vi "Main.vi"(11 "Module Admin":refnum<class "Delacor_lib_QMH_Cloneable Module Admin.lvclass">) -> ()   [LabVIEW 2024, in "Clon.lvlib"]
doc: "This template is based off of the Queued Message Handler design pattern and the Queued Message Handler project template that ships with LabVIEW.\n\nThe main difference is that the queue is private to this module and communication between modules is performed via Broadcast and Request events.\n\nRequest events are wrapped in public API methods and are handled in the Event Handling Loop (EHL) of this VI. Any module can register for Broadcast events sent by this module. The EHL generates messages based on user interface actions.\n\nThe Message Handling Loop (MHL) processes messages generated by the EHL, or by other messages. The messages are string values, so new messages can be added easily to the Message Cases case structure in the MHL. Each message cluster can also provide an optional value for Message Data, which is a variant that can be converted to whatever message-specific data is required.\n_____\nBased on DQMH Dev Tools: Project Template 7.1.0.1503."
uses:
  Clon.lvlib
  <vilib>/Delacor/Delacor QMH/Libraries/Cloneable Module Admin_class/Delacor_lib_QMH_Cloneable Module Admin.lvclass
  Module Data--cluster.ctl
  <vilib>/Delacor/Delacor QMH/Libraries/Message Queue_class/Delacor_lib_QMH_Message Queue.lvclass/Delacor_lib_QMH_Message Queue.ctl
  <vilib>/Delacor/Delacor QMH/Libraries/Cloneable Module Admin_class/Delacor_lib_QMH_Cloneable Module Admin.lvclass/Delacor_lib_QMH_Cloneable Module Admin.ctl
  Stop Argument--cluster.ctl
  <vilib>/Delacor/Delacor QMH/Libraries/Module Admin_class/Delacor_lib_QMH_Module Admin.lvclass/Delacor_lib_QMH_Module Admin.ctl
  Set Volts Argument--cluster.ctl
  <vilib>/Utility/miscctls.llb/LVPointTypeDef.ctl
  <vilib>/Delacor/Delacor QMH/Libraries/Message Queue_class/Delacor_lib_QMH_Enqueue Message (Single).vi
  <vilib>/Delacor/Delacor QMH/Libraries/Cloneable Module Admin_class/Delacor_lib_QMH_Get Module ID.vi
  <vilib>/Delacor/Delacor QMH/Libraries/Module Admin_class/Delacor_lib_QMH_Get External Launch.vi
  <vilib>/Delacor/Delacor QMH/Libraries/Message Queue_class/Delacor_lib_QMH_Message Queue.lvclass
panel:
  out "Meter":dbl(knob) scale=0.0..10.0
  out "error out":errorcluster
  out "Status":string
  in  "Simulate EHL Error":bool
  in  "Simulate MHL Error":bool
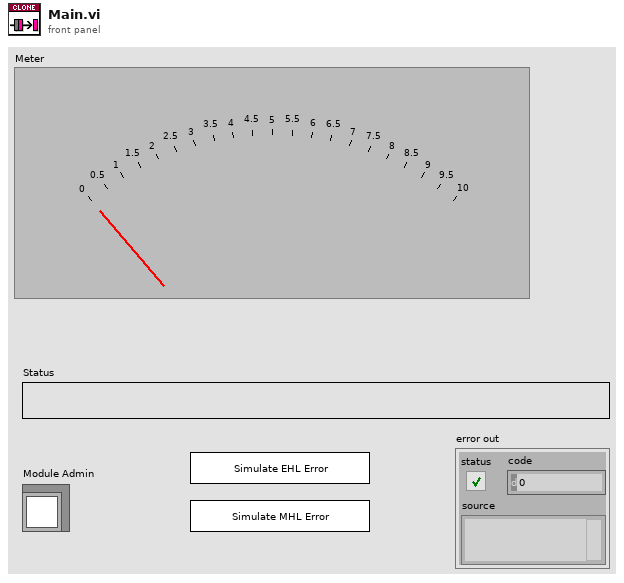
[diagram p1: front panel]
types:
  T1 = typedef "Clon.lvlib/Request Events--cluster.ctl" = cluster{"Stop Module":refnum<user-event>, "Show Panel":refnum<user-event>, "Hide Panel":refnum<user-event>, "Show Diagram":refnum<user-event>, "Get Module Execution Status":refnum<user-event>, "Set Volts":refnum<user-event>}
  T2 = typedef "Clon.lvlib/Module Data--cluster.ctl" = cluster{"Status":string}
  T3 = enum32{"invalid lock state", "Not Locked", "Locked (No Password)", "Password-protected"}
  T4 = typedef "Clon.lvlib/Stop Argument--cluster.ctl" = cluster{"Module ID":i32, "Origin":string, "Exit via Stop Module Req?":bool, "Wait for Module to stop?":bool}
  T5 = typedef "Clon.lvlib/Set Volts Argument--cluster.ctl" = cluster{"Module ID":i32, "Volts":dbl}
  T6 = typedef "LVPointTypeDef.ctl" = cluster{"Horizontal":i16, "Vertical":i16}
  T7 = enum32{"Invalid", "Standard", "Closed", "Hidden", "Minimized", "Maximized"}
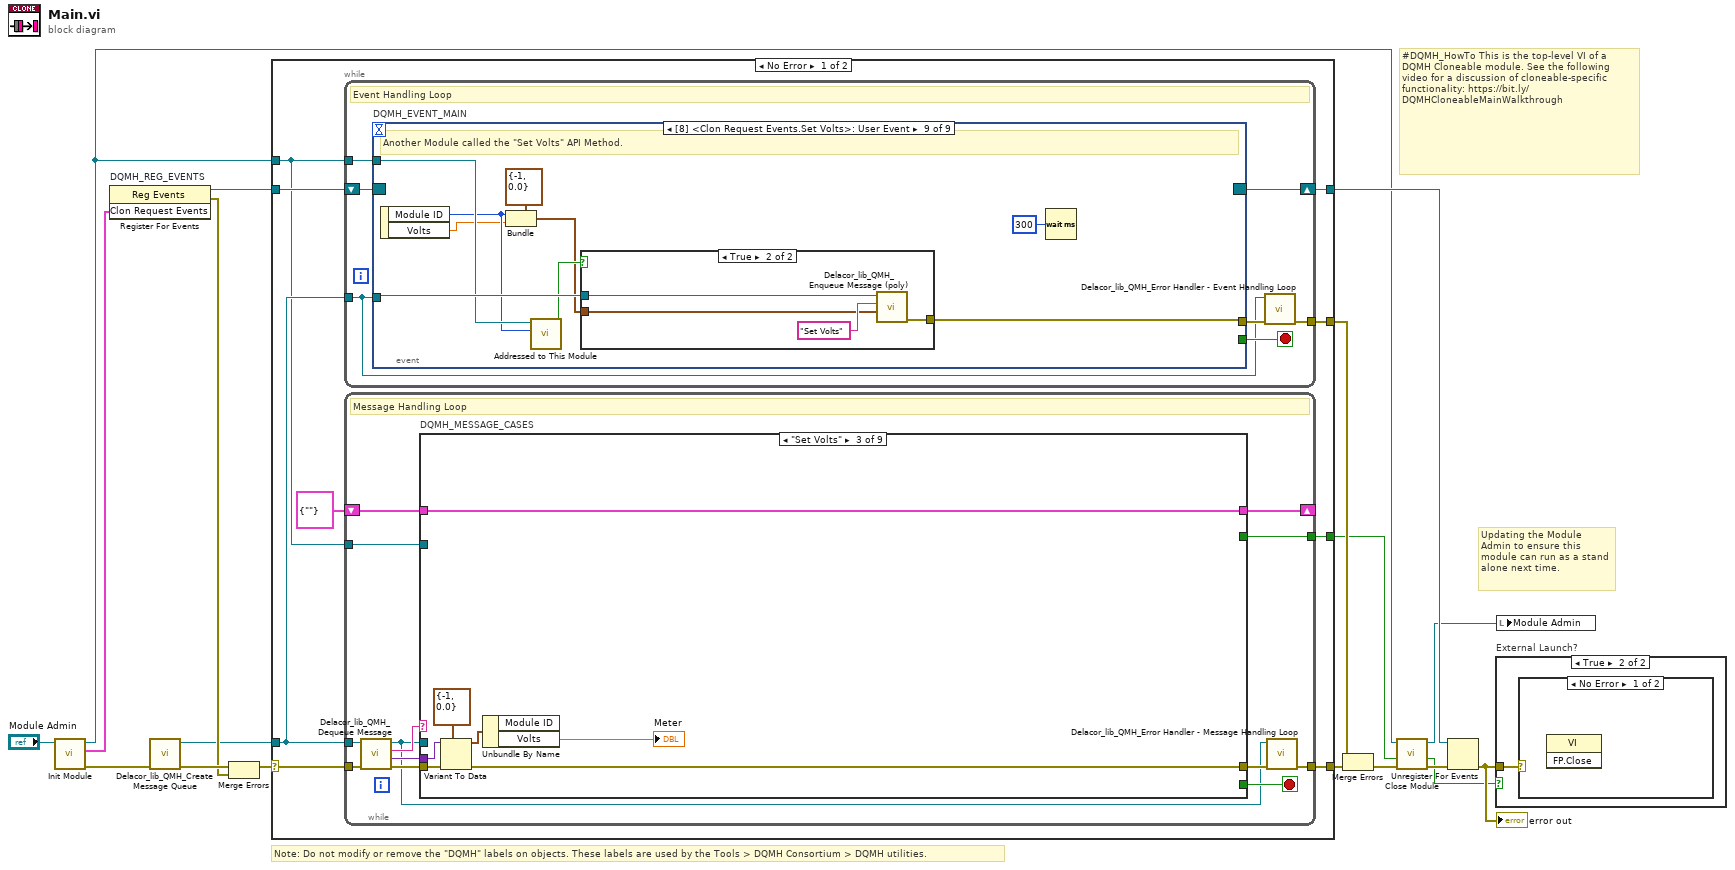
[diagram p0: block diagram]
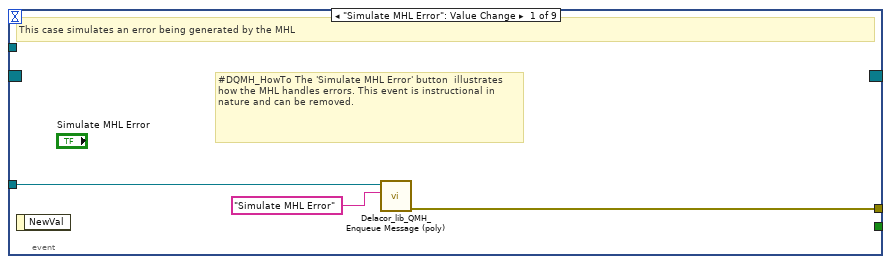
[diagram p2: hidden frame]
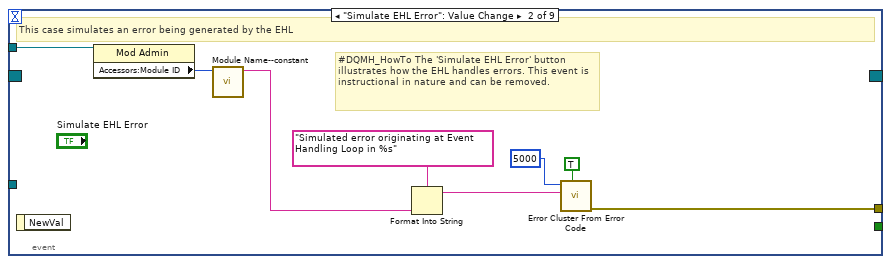
[diagram p3: hidden frame]
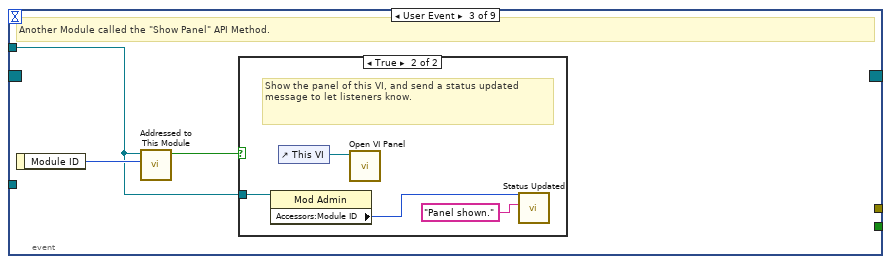
[diagram p4: hidden frame]
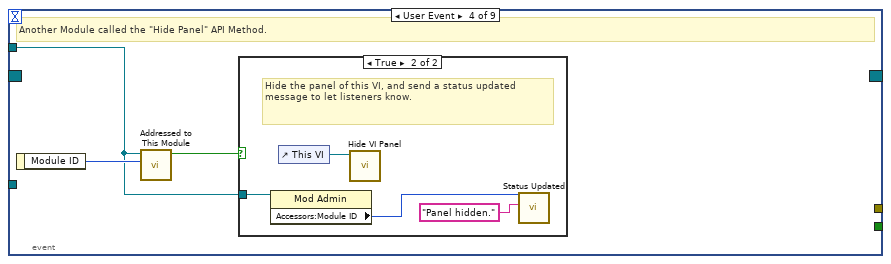
[diagram p6: hidden frame]
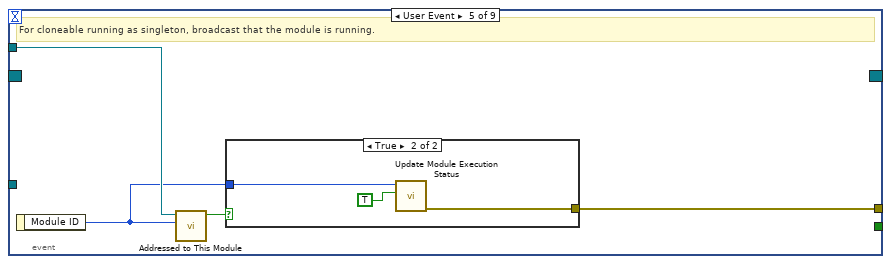
[diagram p8: hidden frame]
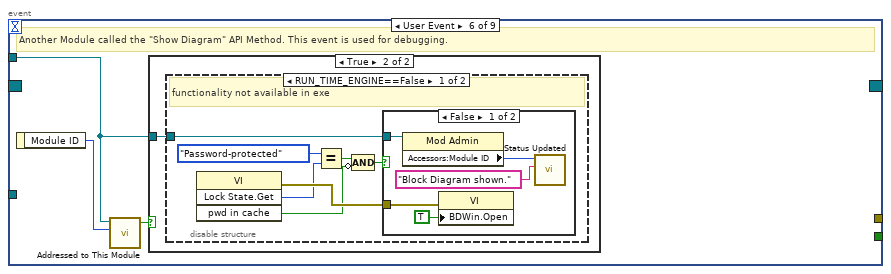
[diagram p10: hidden frame]
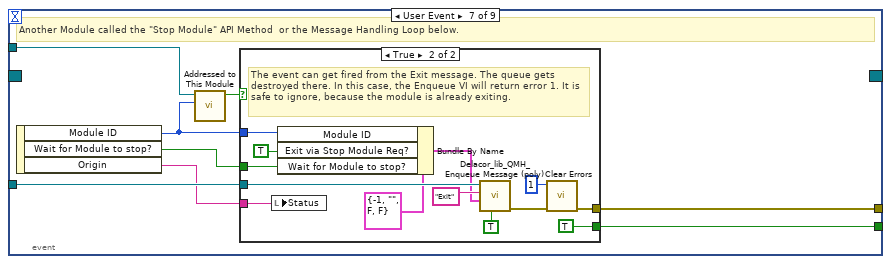
[diagram p14: hidden frame]
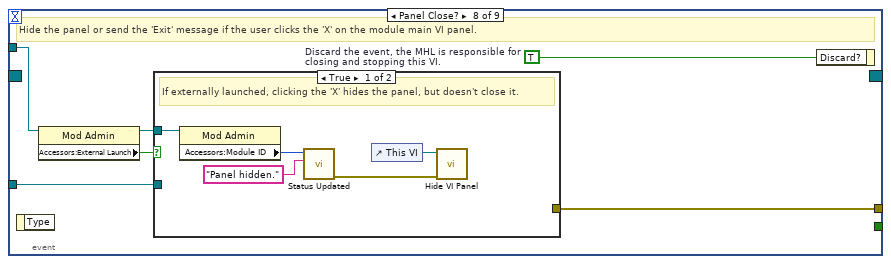
[diagram p16: hidden frame]
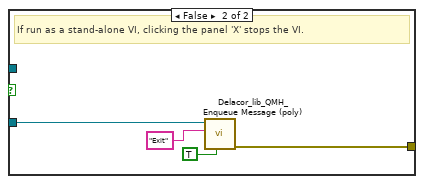
[diagram p17: hidden frame]
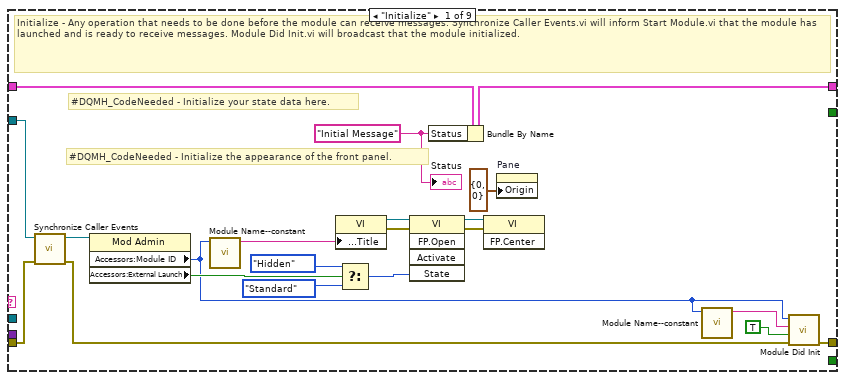
[diagram p19: hidden frame]
diagram:
  # "#DQMH_HowTo This is the top-level VI of a DQMH Cloneable module. See the following video for a discussion of cloneable-specific functionality: https://bit.ly/DQMHCloneableMainWalkthrough"
  # "Note: Do not modify or remove the \"DQMH\" labels on objects. These labels are used by the Tools > DQMH Consortium > DQMH utilities."
  # "Updating the Module Admin to ensure this module can run as a stand alone next time."
  n1 = call "Init Module.vi"("Cloneable Module Admin in"="Module Admin") -> ("error out"=w15:errorcluster, "Clon Request Events"=w7:T1, "Cloneable Module Admin out"=w4:refnum<class "Delacor_lib_QMH_Cloneable Module Admin.lvclass">)  [unwired: 8 in]
  n2 = register-events "DQMH_REG_EVENTS"(w7) -> (reference out=w8:refnum<event-registration>, error out=w10:errorcluster)  [unwired: 2 in]
  n3 = call <vilib>:"Delacor_lib_QMH_Create Message Queue.vi"("error in"=w15) -> ("error out"=w12:errorcluster, "Message Queue"=w6:refnum<class "Delacor_lib_QMH_Message Queue.lvclass">)  [unwired: 9 in]
  n4 = Merge Errors(w12, w10) -> (w11:errorcluster)
  n5 = case shown="No Error" w11 {
    selector: w11 -> [w25 w247]
    tunnel: [w27 w246] -> w16
    tunnel: [w24 w245] -> w9
    tunnel: w8 -> [w22 w245]
    tunnel: w6 -> [w21 w238]
    tunnel: [w26 _] -> w17
    tunnel: w4 -> [w20 w241]
    tunnel: [w19 _] -> w2
    frame No Error {
      n6 = while {
        tunnel: w21 -> [w28]
        shift-right: [w31] -> w24
        shift-left: w22 -> [w32]
        tunnel: [w33] -> w26
        tunnel: w20 -> [w29]
        stop <- w30 stop-if-true
        # "Event Handling Loop"
        n7 = event "DQMH_EVENT_MAIN" shown="[8] <Clon Request Events.Set Volts>: User Event" {
          selector: w32 -> [_ _ _ _ _ _ _ _ _]
          dyn-events: [_ _ _ _ _ _ _ _ _] -> w31
          timeout: _ -> [_ _ _ _ _ _ _ _ _]
          tunnel: [_ _ _ _ _ _ w86 _ _] -> w30
          tunnel: w28 -> [w36 _ _ _ _ _ w89 w106 w127]
          tunnel: [w37 w45 _ _ w63 _ w90 w109 w120] -> w34
          tunnel: w29 -> [_ w44 w46 w53 w61 w67 w88 w107 w125]
          event "Simulate MHL Error": Value Change {
            # "#DQMH_HowTo The 'Simulate MHL Error' button  illustrates how the MHL handles errors. This event is instructional in nature and can be removed."
            # "This case simulates an error being generated by the MHL"
            n8 = event-data() -> ()  [unwired: 1 in, 1 out]
            n9 = call-poly <vilib>:"Delacor_lib_QMH_Enqueue Message (poly).vi"("Message"="Simulate MHL Error", "Message Queue in"=w36) -> ("error out"=w37:errorcluster)  [unwired: 8 in, 1 out]
          }
          event "Simulate EHL Error": Value Change {
            # "#DQMH_HowTo The 'Simulate EHL Error' button  illustrates how the EHL handles errors. This event is instructional in nature and can be removed."
            # "This case simulates an error being generated by the EHL"
            n10 = event-data() -> ()  [unwired: 1 in, 1 out]
            n11 = property on="Property Node" class="Mod Admin"(reference=w44) -> ("Accessors:Module ID"=w43:i32)  [unwired: 1 in, 2 out]
            n12 = call "Module Name--constant.vi"("Module ID"=w43) -> ("Module Name"=w38:string)  [unwired: 10 in]
            n13 = Format Into String(format string="Simulated error originating at Event Handling Loop in %s", w38) -> (resulting string=w41:string)  [unwired: 2 in, 1 out]
            n14 = call <vilib>:"Error Cluster From Error Code.vi"("show call chain? (False)"=TRUE, "error message (\"\")"=w41, "error code (0)"=5000) -> ("error out"=w45:errorcluster)  [unwired: 6 in]
          }
          event User Event {
            # "Another Module called the \"Show Panel\" API Method."
            n15 = event-data() -> ("Module ID"=w47:i32)  [unwired: 1 in]
            n16 = call "Addressed to This Module.vi"("Module ID from Argument"=w47, "Module Admin"=w46) -> ("Addressed to this instance?"=w48:bool)  [unwired: 8 in, 1 out]
            n17 = case shown="True" w48 {
              tunnel: w46 -> [_ w50]
              frame False {
              }
              frame True {
                # "Show the panel of this VI, and send a status updated message to let listeners know."
                n18 = property on="Property Node" class="Mod Admin"(reference=w50) -> ("Accessors:Module ID"=w49:i32)  [unwired: 1 in, 2 out]
                n19 = control-ref of="This VI"() -> (w52:refnum<vi>)
                n20 = call "Open VI Panel.vi"("VI"=w52) -> ()  [unwired: 10 in, 1 out]
                n21 = call "Status Updated.vi"("Status"="Panel shown." ("format string"), "Module ID"=w49) -> ()  [unwired: 9 in, 1 out]
              }
            }
          }
          event User Event {
            # "Another Module called the \"Hide Panel\" API Method."
            n22 = event-data() -> ("Module ID"=w54:i32)  [unwired: 1 in]
            n23 = call "Addressed to This Module.vi"("Module ID from Argument"=w54, "Module Admin"=w53) -> ("Addressed to this instance?"=w55:bool)  [unwired: 8 in, 1 out]
            n24 = case shown="True" w55 {
              tunnel: w53 -> [_ w57]
              frame False {
              }
              frame True {
                # "Hide the panel of this VI, and send a status updated message to let listeners know."
                n25 = property on="Property Node" class="Mod Admin"(reference=w57) -> ("Accessors:Module ID"=w56:i32)  [unwired: 1 in, 2 out]
                n26 = control-ref of="This VI"() -> (w59:refnum<vi>)
                n27 = call "Hide VI Panel.vi"("VI"=w59) -> ()  [unwired: 10 in, 1 out]
                n28 = call "Status Updated.vi"("Status"="Panel hidden." ("format string"), "Module ID"=w56) -> ()  [unwired: 9 in, 1 out]
              }
            }
          }
          event User Event {
            # "For cloneable running as singleton, broadcast that the module is running."
            n29 = event-data() -> ("Module ID"=w60:i32)  [unwired: 1 in]
            n30 = call "Addressed to This Module.vi"("Module ID from Argument"=w60, "Module Admin"=w61) -> ("Addressed to this instance?"=w62:bool)  [unwired: 8 in, 1 out]
            n31 = case shown="True" w62 {
              tunnel: [_ w66] -> w63
              tunnel: w60 -> [_ w65]
              frame False {
              }
              frame True {
                n32 = call "Update Module Execution Status.vi"("Running?"=TRUE, "Module ID"=w65) -> ("error out"=w66:errorcluster)  [unwired: 9 in]
              }
            }
          }
          event User Event {
            # "Another Module called the \"Show Diagram\" API Method. This event is used for debugging."
            n33 = event-data() -> ("Module ID"=w68:i32)  [unwired: 1 in]
            n34 = call "Addressed to This Module.vi"("Module ID from Argument"=w68, "Module Admin"=w67) -> ("Addressed to this instance?"=w69:bool)  [unwired: 8 in, 1 out]
            n35 = case shown="True" w69 {
              tunnel: w67 -> [_ w70]
              frame False {
              }
              frame True {
                n36 = disable-structure shown="RUN_TIME_ENGINE==False" {
                  disable-tunnel: w70 -> [w71 _]
                  frame condition #0 (active) {
                    # "functionality not available in exe"
                    n37 = invoke on="Invoke Node" class="VI" method="Lock State.Get"() -> (error out=w77:errorcluster, "Get Lock State"=w76:T3, "pwd in cache"=w73:bool)  [unwired: 4 in, 1 out]
                    n38 = Equal?(x=T3."Password-protected", y=w76) -> (x = y?=w74:bool)
                    n39 = Compound Arithmetic op=AND(w74, invert w73) -> (w72:bool)
                    n40 = case shown="False" w72 {
                      tunnel: w77 -> [w82 _]
                      tunnel: w71 -> [w79 _]
                      frame False {
                        n41 = property on="Property Node" class="Mod Admin"(reference=w79) -> ("Accessors:Module ID"=w78:i32)  [unwired: 1 in, 2 out]
                        n42 = property on="Property Node" class="VI"(error in=w82, "BDWin.Open"=TRUE ("Block Diagram Window:Open")) -> ()  [unwired: 1 in, 2 out]
                        n43 = call "Status Updated.vi"("Status"="Block Diagram shown." ("format string"), "Module ID"=w78) -> ()  [unwired: 9 in, 1 out]
                      }
                      frame True {
                        # "Password-protected VI, and the password is not in the cache. Do not show the diagram."
                      }
                    }
                  }
                  frame condition #1 {
                  }
                }
              }
            }
          }
          event User Event {
            # "Another Module called the \"Stop Module\" API Method  or the Message Handling Loop below."
            n44 = event-data() -> ("Module ID"=w84:i32, "Wait for Module to stop?"=w85:bool, "Origin"=w83:string)  [unwired: 1 in]
            n45 = call "Addressed to This Module.vi"("Module ID from Argument"=w84, "Module Admin"=w88) -> ("Addressed to this instance?"=w87:bool)  [unwired: 8 in, 1 out]
            n46 = case shown="True" w87 {
              tunnel: [_ w102] -> w90
              tunnel: w89 -> [_ w98]
              tunnel: [_ TRUE] -> w86
              tunnel: w85 -> [_ w93]
              tunnel: w84 -> [_ w95]
              tunnel: w83 -> [_ w91]
              frame False {
              }
              frame True {
                # "The event can get fired from the Exit message. The queue gets destroyed there. In this case, the Enqueue VI will return error 1. It is safe to ignore, because the module is already exiting."
                n47 = local write "Status"(w91) -> ()
                n48 = Bundle By Name(cluster=T4 {"Module ID"=-1, "Origin"="", "Exit via Stop Module Req?"=FALSE, "Wait for Module to stop?"=FALSE} ("Stop Argument"), "Module ID"=w95, "Exit via Stop Module Req?"=TRUE, "Wait for Module to stop?"=w93) -> (w92:T4)
                n49 = call-poly <vilib>:"Delacor_lib_QMH_Enqueue Message (poly).vi"("Priority Message? (F)"=TRUE, "Message Data"=w92, "Message"="Exit", "Message Queue in"=w98) -> ("error out"=w103:errorcluster)  [unwired: 6 in, 1 out]
                n50 = call <vilib>:"Clear Errors.vi"("error in (no error)"=w103, "specific error code to clear (0: all)"=1) -> ("error out"=w102:errorcluster)  [unwired: 4 in, 1 out]
              }
            }
          }
          event Panel Close? {
            w108 = TRUE  # Discard the event, the MHL is responsible for closing and stopping this VI.
            # "Hide the panel or send the 'Exit' message if the user clicks the 'X' on the module main VI panel."
            n51 = event-data() -> ()  [unwired: 1 in, 1 out]
            n52 = property on="Property Node" class="Mod Admin"(reference=w107) -> (reference out=w104:refnum<class "Delacor_lib_QMH_Cloneable Module Admin.lvclass">, "Accessors:External Launch"=w105:bool)  [unwired: 1 in, 1 out]
            n53 = case shown="True" w105 {
              tunnel: w106 -> [_ w117]
              tunnel: [_ w118] -> w109
              tunnel: w104 -> [w112 _]
              frame True {
                # "If externally launched, clicking the 'X' hides the panel, but doesn't close it."
                n54 = property on="Property Node" class="Mod Admin"(reference=w112) -> ("Accessors:Module ID"=w111:i32)  [unwired: 1 in, 2 out]
                n55 = call "Status Updated.vi"("Status"="Panel hidden." ("format string"), "Module ID"=w111) -> ("error out"=w110:errorcluster)  [unwired: 9 in]
                n56 = control-ref of="This VI"() -> (w114:refnum<vi>)
                n57 = call "Hide VI Panel.vi"("error in"=w110, "VI"=w114) -> ()  [unwired: 9 in, 1 out]
              }
              frame False {
                # "If run as a stand-alone VI, clicking the panel 'X' stops the VI."
                n58 = call-poly <vilib>:"Delacor_lib_QMH_Enqueue Message (poly).vi"("Priority Message? (F)"=TRUE, "Message"="Exit", "Message Queue in"=w117) -> ("error out"=w118:errorcluster)  [unwired: 7 in, 1 out]
              }
            }
            n59 = event-data ("Event Filter Node")("Discard?"=w108) -> ()  [unwired: 1 in, 1 out]
          }
          event User Event {
            # "Another Module called the \"Set Volts\" API Method."
            n60 = event-data() -> ("Module ID"=w122:i32, "Volts"=w121:dbl)  [unwired: 1 in]
            n61 = Bundle(cluster=T5 {"Module ID"=-1, "Volts"=0.0} ("Set Volts Argument"), "Module ID"=w122, "Volts"=w121) -> (w123:T5)
            n62 = call "Addressed to This Module.vi"("Module ID from Argument"=w122, "Module Admin"=w125) -> ("Addressed to this instance?"=w126:bool)  [unwired: 8 in, 1 out]
            n63 = case shown="True" w126 {
              tunnel: w127 -> [_ w131]
              tunnel: w123 -> [_ w129]
              tunnel: [_ w128] -> w120
              frame False {
              }
              frame True {
                n64 = call-poly <vilib>:"Delacor_lib_QMH_Enqueue Message (poly).vi"("Message Data"=w129, "Message"="Set Volts", "Message Queue in"=w131) -> ("error out"=w128:errorcluster)  [unwired: 7 in, 1 out]
              }
            }
            n65 = Wait (ms)(milliseconds to wait=u32 300) -> ()  [unwired: 1 out]
          }
        }
        n66 = call-dynamic "Delacor_lib_QMH_Error Handler - Event Handling Loop.vi"("error in"=w34, "Message Queue in"=w28) -> ("dup error in"=w33:errorcluster)  [unwired: 8 in, 1 out]
      }
      n67 = while {
        tunnel: w21 -> [w132]
        shift-right: [w139] -> _
        shift-left: T2 {"Status"=""} ("Data Cluster") -> [w140]
        tunnel: w25 -> [w143]
        tunnel: [w141] -> w27
        tunnel: w20 -> [w134]
        tunnel: [w133] -> w19
        stop <- w138 stop-if-true
        # "Message Handling Loop"
        n68 = call-dynamic "Delacor_lib_QMH_Dequeue Message.vi"("error in"=w143, "Message Queue in"=w132) -> ("error out"=w142:errorcluster, "Message Data"=w136:variant, "Message"=w137:string, "Message Queue out"=w135:refnum<class "Delacor_lib_QMH_Message Queue.lvclass">)  [unwired: 6 in]
        n69 = case "DQMH_MESSAGE_CASES" shown="\"Set Volts\"" w137 {
          selector: w137 -> [_ _ _ _ _ _ _ _ w227]
          tunnel: w135 -> [_ _ _ _ _ w182 _ w219 _]
          tunnel: w142 -> [w163 w167 w174 w177 w179 w191 w208 w225 w236]
          tunnel: [w161 w167 w172 w176 w179 w187 w207 w220 w237] -> w144
          tunnel: w140 -> [w154 w166 w173 w175 w178 w186 w205 w218 w234]
          tunnel: [w153 w166 w173 w175 w178 w186 w205 w218 w234] -> w139
          tunnel: [_ _ _ _ _ _ _ w217 _] -> w138
          tunnel: w136 -> [_ _ w171 _ _ w185 _ w215 _]
          tunnel: w134 -> [w149 _ _ _ _ w184 w203 w210 w233]
          tunnel: [_ _ _ _ _ _ _ w213 _] -> w133
          frame "Initialize" {
            w146 = "Initial Message" ("Initial Message")
            # "#DQMH_CodeNeeded - Initialize the appearance of the front panel."
            # "#DQMH_CodeNeeded - Initialize your state data here."
            # "Initialize - Any operation that needs to be done before the module can receive messages. Synchronize Caller Events.vi will inform Start Module.vi that the module has launched and is ready to receive messages. Module Did Init.vi will broadcast that the module initialized."
            n70 = call "Synchronize Caller Events.vi"("error in"=w163, "Module Admin"=w149) -> ("error out"=w162:errorcluster, "Module Admin out"=w148:refnum<class "Delacor_lib_QMH_Cloneable Module Admin.lvclass">)  [unwired: 8 in]
            n71 = property on="Property Node" class="Mod Admin"(reference=w148) -> ("Accessors:Module ID"=w145:i32, "Accessors:External Launch"=w150:bool)  [unwired: 1 in, 2 out]
            n72 = call "Module Name--constant.vi"("Module ID"=w145) -> ("Module Name"=w158:string)  [unwired: 10 in]
            n73 = property on="Property Node" class="VI"("Front Panel.Title"=w158) -> (reference out=w160:refnum<vi>, error out=w165:errorcluster)  [unwired: 2 in]
            n74 = Select(t=T7."Hidden" ("State"), s=w150, f=T7."Standard" ("State")) -> (s? t:f=w155:T7)
            n75 = invoke on="Invoke Node" class="VI" method="FP.Open"(reference=w160, error in=w165, "State"=w155) -> (reference out=w159:refnum<vi>, error out=w164:errorcluster)  [unwired: 2 in, 3 out]
            n76 = Bundle By Name(cluster=w154, "Status"=w146) -> (w153:T2)
            n77 = invoke on="Invoke Node" class="VI" method="FP.Center"(reference=w159, error in=w164) -> ()  [unwired: 1 in, 3 out]
            n78 = property on="Pane" class="Pane"("Origin"=T6 {"Horizontal"=0, "Vertical"=0}) -> ()  [unwired: 2 in, 2 out]
            n79 = call "Module Name--constant.vi"("Module ID"=w145) -> ("Module Name"=w151:string)  [unwired: 10 in]
            n80 = call "Module Did Init.vi"("error in"=w162, "Initialized?"=TRUE, "Origin"=w151, "Module ID"=w145) -> ("error out"=w161:errorcluster)  [unwired: 7 in]
            "Status" <- w146
          }
          frame "---Module Specific---" {
            # "Separator -- The following cases handle messages specific to this Module."
          }
          frame "Set Volts" {
            n81 = Variant To Data(error in=w174, type=T5 {"Module ID"=-1, "Volts"=0.0} ("Set Volts Argument"), Variant=w171) -> (data=w169:T5, error out=w172:errorcluster)
            n82 = Unbundle By Name(w169) -> ("Volts"=→"Meter":dbl)  [unwired: 1 out]
          }
          frame "---Copy This Frame---" {
            # "Duplicate this frame when creating new messages.  Change this comment in the duplicated frame to describe this message."
            n83 = Merge Errors(w177) -> (w176:errorcluster)
          }
          frame "---Exit and Error Handling---" {
            # "Separator - the following cases handle errors and exit messages."
          }
          frame "Error" {
            # "#DQMH_CodeRecommended - If the module is running in standalone mode (External Launch = FALSE), this code will pop up an error dialog and call the 'Exit' message if an error occurs. Add more fine-grained error management here."
            # "Error - Check the error message data and respond accordingly. This message is sent by the \"Error Handler\" VIs at the end of each loop in this application."
            n84 = property on="Property Node" class="Mod Admin"(reference=w184) -> ("Accessors:External Launch"=w183:bool, "Accessors:Module ID"=w181:i32)  [unwired: 1 in, 2 out]
            n85 = Variant To Data(error in=w191, type=errorcluster {"status"=FALSE, "code"=0, "source"=""} ("error constant"), Variant=w185) -> (data=w180:errorcluster, error out=w189:errorcluster)
            n86 = local write "error out"(w180) -> ()
            n87 = call "Error Reported.vi"("Error"=w180, "Module ID"=w181) -> ()  [unwired: 9 in, 1 out]
            n88 = case shown="False" w183 {
              tunnel: [w196 _] -> w188
              tunnel: w182 -> [w194 _]
              tunnel: w180 -> [w195 _]
              frame False {
                n89 = disable-structure shown="Default" {
                  disable-tunnel: w195 -> [w197 _]
                  frame condition #0 (active) {
                    # "If the module is running standalone, then pop up an error dialog and call the \"Exit\" message."
                    n90 = call <vilib>:"Simple Error Handler.vi"("error in (no error)"=w197) -> ()  [unwired: 4 in, 5 out]
                  }
                  frame condition #1 {
                    # "To prevent the Simple Error Handler VI from being loaded (e.g. when deploying to a Real-Time target), add the Conditional Disable Symbol \"DQMH_Disable_SEH\" to your project and set it to TRUE."
                  }
                }
                n91 = call-poly <vilib>:"Delacor_lib_QMH_Enqueue Message (poly).vi"("Priority Message? (F)"=TRUE, "Message"="Exit", "Message Queue in"=w194) -> ("error out"=w196:errorcluster)  [unwired: 7 in, 1 out]
              }
              frame True {
                # "If the module was launched externally, calling the Error Reported broadcast VI is the only action performed by the \"Error\" message. The module's caller can then process the error appropriately."
              }
            }
            n92 = Merge Errors(w189, w188) -> (w187:errorcluster)
          }
          frame "Simulate MHL Error" {
            # "#DQMH_HowTo The 'Simulate MHL Error' button  illustrates how the MHL handles errors. This event is instructional in nature and can be removed."
            # "Simulate an error occurring at the MHL"
            n93 = property on="Property Node" class="Mod Admin"(reference=w203) -> ("Accessors:Module ID"=w204:i32)  [unwired: 1 in, 2 out]
            n94 = call "Module Name--constant.vi"("Module ID"=w204) -> ("Module Name"=w199:string)  [unwired: 10 in]
            n95 = Format Into String(format string="Simulated error originating at Message Handling Loop in %s", w199) -> (resulting string=w200:string)  [unwired: 2 in, 1 out]
            n96 = call <vilib>:"Error Cluster From Error Code.vi"("show call chain? (False)"=TRUE, "error message (\"\")"=w200, "error code (0)"=5001) -> ("error out"=w206:errorcluster)  [unwired: 6 in]
            n97 = Merge Errors(w208, w206) -> (w207:errorcluster)
          }
          frame "Exit" {
            w216 = 91  # 91: not all Exit messages will have an argument
            w217 = TRUE  # Stop the VI
            # "Release the message queue reference"
            # "#DQMH_CodeNeeded - Add any required cleanup code here."
            # "Exit - Exit the application."
            n98 = Variant To Data(error in=w225, type=T4 {"Module ID"=-1, "Origin"="", "Exit via Stop Module Req?"=FALSE, "Wait for Module to stop?"=FALSE} ("Stop Argument"), Variant=w215) -> (data=w212:T4, error out=w221:errorcluster)
            n99 = call <vilib>:"Clear Errors.vi"("error in (no error)"=w221, "specific error code to clear (0: all)"=w216) -> ("error out"=w224:errorcluster)  [unwired: 4 in, 1 out]
            n100 = property on="Property Node" class="Mod Admin"(reference=w210) -> ("Accessors:Module ID"=w209:i32)  [unwired: 1 in, 2 out]
            n101 = control-ref of="This VI"() -> (w211:refnum<vi>)
            n102 = call-dynamic "Delacor_lib_QMH_Release Message Queue.vi"("error in"=w224, "Message Queue"=w219) -> ("error out"=w223:errorcluster)  [unwired: 9 in]
            n103 = call "Handle Exit.vi"("Stop Argument"=w212, "Module Admin in"=w210, "VI reference"=w211) -> ("error out"=w222:errorcluster, "Wait for Stop?"=w213:bool)  [unwired: 7 in]
            n104 = Merge Errors(w223, w222) -> (w220:errorcluster)
            n105 = call "Error Reported.vi"("Error"=w220, "Module ID"=w209) -> ()  [unwired: 9 in, 1 out]
          }
          frame Default {
            # "'Default' case only runs if there is a message that isn't defined in any of the other cases.  Output a programming error."
            n106 = property on="Property Node" class="Mod Admin"(reference=w233) -> ("Accessors:Module ID"=w232:i32)  [unwired: 1 in, 2 out]
            n107 = call "Module Name--constant.vi"("Module ID"=w232) -> ("Module Name"=w226:string)  [unwired: 10 in]
            n108 = Format Into String(format string="The invalid message string \"%s\" was received in the Message Handling Loop for module \"%s\".", w227, w226) -> (resulting string=w229:string)  [unwired: 2 in, 1 out]
            n109 = call <vilib>:"Error Cluster From Error Code.vi"("show call chain? (False)"=TRUE, "error message (\"\")"=w229, "error code (0)"=1) -> ("error out"=w235:errorcluster)  [unwired: 6 in]
            n110 = Merge Errors(w236, w235) -> (w237:errorcluster)
          }
        }
        n111 = call-dynamic "Delacor_lib_QMH_Error Handler - Message Handling Loop.vi"("error in"=w144, "Message Queue in"=w135) -> ("dup error in"=w141:errorcluster)  [unwired: 8 in, 1 out]
      }
    }
    frame Error {
      n112 = call "Synchronize Caller Events.vi"("Module Admin"=w241) -> ("Module Admin out"=w240:refnum<class "Delacor_lib_QMH_Cloneable Module Admin.lvclass">)  [unwired: 9 in, 1 out]
      n113 = property on="Property Node" class="Mod Admin"(reference=w240) -> ("Accessors:Module ID"=w239:i32)  [unwired: 1 in, 2 out]
      n114 = call-dynamic "Delacor_lib_QMH_Release Message Queue.vi"("error in"=w247, "Message Queue"=w238) -> ("error out"=w246:errorcluster)  [unwired: 9 in]
      n115 = call "Module Name--constant.vi"("Module ID"=w239) -> ("Module Name"=w244:string)  [unwired: 10 in]
      n116 = Format Into String(format string="An error occurred during initialization. %s is no longer running.", w244) -> (resulting string=w242:string)  [unwired: 2 in, 1 out]
      n117 = call "Error Reported.vi"("Additional Information"=w242, "Error"=w246, "Module ID"=w239) -> ()  [unwired: 8 in, 1 out]
    }
  }
  n118 = Merge Errors(w17, w16) -> (w18:errorcluster)
  n119 = call "Close Module.vi"("error in"=w18, "Wait for stop?"=w2, "Module Admin in"=w4) -> ("error out"=w14:errorcluster, "External Launch"=w1:bool, "Module Admin out"=w3:refnum<class "Delacor_lib_QMH_Cloneable Module Admin.lvclass">)  [unwired: 6 in]
  n120 = Unregister For Events(event registration refnum=w9, error in=w14) -> (error out=w13:errorcluster)
  "error out" <- w13
  n121 = case "External Launch?" shown="True" w1 {
    tunnel: w13 -> [_ w248]
    frame False {
    }
    frame True {
      n122 = case shown="No Error" w248 {
        frame No Error {
          n123 = invoke class="VI" method="FP.Close"() -> ()  [unwired: 3 in, 3 out]
        }
        frame Error {
          n124 = disable-structure shown="Default" {
            frame condition #0 (active) {
              n125 = invoke class="VI" method="FP.Open"("Activate"=TRUE ("Activate?")) -> ()  [unwired: 4 in, 5 out]
            }
            frame condition #1 {
              # "Don't show panel on error if running inside a built EXE."
            }
          }
        }
      }
    }
  }
  n126 = local write "Module Admin"(w3) -> ()
